vi "RecrystalliseTCPcomm.vi"(8 "error in (no error)":errorcluster, 11 "DC voltage in":i32) -> (0 "error out":errorcluster)   [LabVIEW 2019]
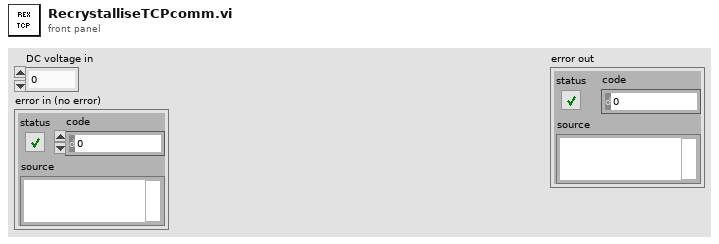
[diagram p1: front panel]
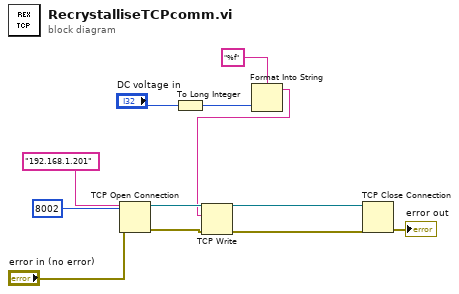
[diagram p0: block diagram]
diagram:
  n1 = TCP Open Connection(address="192.168.1.201", remote port or service name=u16 8002, error in (no error)="error in (no error)") -> (connection ID=w10:refnum<k5>, error out=w3:errorcluster)  [unwired: 2 in]
  n2 = To Long Integer(number="DC voltage in") -> (32bit integer=w5:i32)
  n3 = Format Into String(format string="%f", w5) -> (resulting string=w4:string)  [unwired: 2 in, 1 out]
  n4 = TCP Write(connection ID=w10, data in=w4, error in (no error)=w3) -> (connection ID out=w8:refnum<k5>, error out=w7:errorcluster)  [unwired: 1 in, 1 out]
  n5 = TCP Close Connection(connection ID=w8, error in (no error)=w7) -> (error out=→"error out":errorcluster)  [unwired: 1 in, 1 out]
